vi "Read PID.vi"(7 "PIDs":T1, 8 "error in (no error)":errorcluster, 11 "VISA Refnum in":refnum<visa-resource-name>) -> (0 "error out":errorcluster, 2 "Response":string, 3 "Result":dbl format="%.2f")   [LabVIEW 2011]
uses:
  PID List.ctl
panel:
  out "number":u16
  out "length 2":i32
  out "sum":u32
  out "length":i32
  out "Serial Settings:Number of Bytes at Serial Port":u32
  out "read buffer 2":string
  out "read buffer":string
  out "Array":string[](array[string])
  out "Responses":string[](array[string])
  out "VISA Refnum in 2":refnum<visa-resource-name>
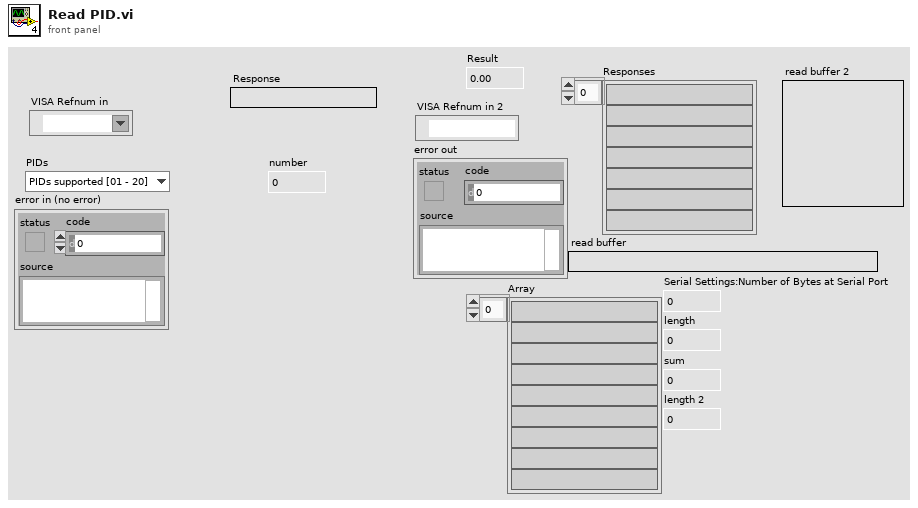
[diagram p1: front panel]
types:
  T1 = typedef "PID List.ctl" = enum16{"PIDs supported [01 - 20]", "Monitor status since DTCs cleared", "Freeze DTC", "Fuel system status", "Caulculated engine load value", "Engine Coolant temperature", "Short term fuel %trim Bank1", "Long term fuel %trim Bank 1", "Short term fuel %trim Bank2", "Long term fuel %trim Bank2", "Fuel pressure", "Intake manifold absolute pressure", "Engine RPM", "Vehicle speed", "timing advance", "Intake air temperature", "MAF air flow rate", "Throttle position", "Commanded secondary air status", "Oxygen sensors present", "bank 1 sensor 1", "Bank 1 sensor 2", "Bank 1 sensor 3", "Bank 1 sensor 4", "Bank 2 sensor 1", "Bank 2 sensor 2", "Bank 2 sensor 3", "Bank 2 sensor 4", "OBD standards this vehicle conforms to", "Oxygen sensor present", "Auxilary input status", "Run time since engine start", "PIDs supported [21-40]", "Distance traveled with malfunction", "Fuel Rail Pressure (manifold)", "Fuel Rail Pressure (gasoline)", "O2S1_WR", "O2S2_WR", "O2S3_WR", "O2S4_WR", "O2S5_WR", "O2S6_WR", "O2S7_WR", "O2S8_WR", "Commanded EGR", "EGR Error", "Commanded evaporative purge", "Fuel Level Input", "# of warm ups since codes cleared", "Distance traveled since codes cleared", "Evap System Vapor Pressure", "Barometric pressure", "O2S1", "O2S2", "O2S3", "O2S4", "O2S5", "O2S6", "O2S7", "O2S8", "Catalyst Temperature B1S1", "Catalyst Temperature B2S1", "Catalyst Temperature B1S2", "Catalyst Temperature B2S2", "PIDs supported [41-60]", "Monitor status this drive cycle", "Control module voltage", "Absolute load value", "Command equivalence ratio", "Relative throttle position", "Ambient air temperature", "Absolute throttle position B", "Absolute throttle position C", "Accelerator pedal position D", "Accelerator pedal position E", "Accelerator pedal position F", "Command throttle actuator", "PIDs supported [61-80]", "Auxilary input / output supported", "Mass air flow sensor", "Engine coolant temperature", "Intake air temperature sensor", "Commanded EGR and EGR Error", "Fuel pressure control system", "Injection pressure control system", "Turbocharger compressor inlet pressure", "Boost pressure control", "Exhaust pressure", "Turbocharger RPM", "Turbocharger temperature", "Turbocharger temperature2", "Vehicle Identification number (VIN)"}
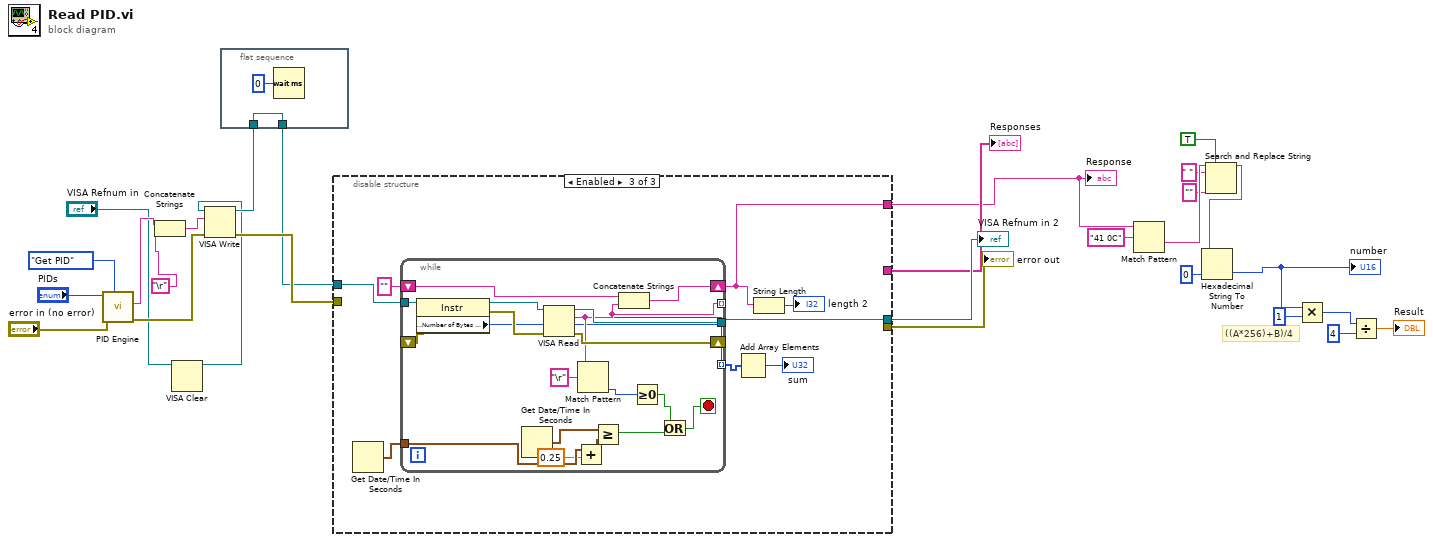
[diagram p0: block diagram]
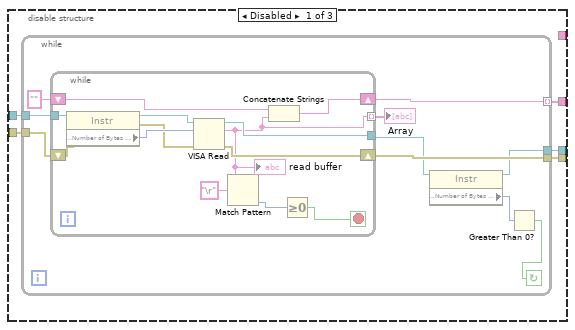
[diagram p2: hidden frame]
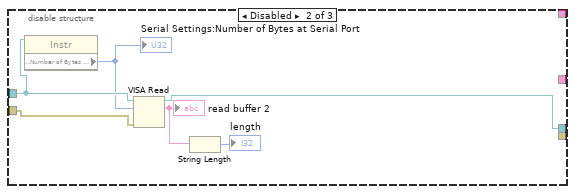
[diagram p3: hidden frame]
diagram:
  # "((A*256)+B)/4"
  n1 = call "PID Engine.vi"("State"=enum16{"Init", "Get PID"}."Get PID", "error in (no error)"="error in (no error)", "PIDs"="PIDs") -> ("error out"=w25:errorcluster, "String"=w22:string)  [unwired: 5 in, 2 out]
  n2 = Concatenate Strings(w22, "\r") -> (w21:string)
  n3 = VISA Clear(VISA resource name="VISA Refnum in") -> (VISA resource name out=w14:refnum<visa-resource-name>)  [unwired: 1 in, 1 out]
  n4 = VISA Write(VISA resource name=w14, write buffer=w21, error in (no error)=w25) -> (VISA resource name out=w16:refnum<visa-resource-name>, error out=w24:errorcluster)  [unwired: 1 out]
  n5 = flat-sequence {
    tunnel: [w29] -> w17
    tunnel: w16 -> [w29]
    frame #0 {
      n6 = Wait (ms)(milliseconds to wait=u32 0) -> ()  [unwired: 1 out]
    }
  }
  n7 = disable-structure shown="Enabled" {
    disable-tunnel: w24 -> [w35 w64 _]
    disable-tunnel: [w34 _ _] -> w23
    disable-tunnel: [w33 w63 w66] -> w19
    disable-tunnel: [w32 _ _] -> w18
    disable-tunnel: w17 -> [w31 w62 w71]
    disable-tunnel: [_ _ w67] -> w13
    frame Disabled {
      n8 = while {
        tunnel: w31 -> [w45]
        tunnel: [w43] -> w32 mode=indexing
        tunnel: w35 -> [w42]
        tunnel: [w41] -> w34
        tunnel: [w39] -> w33
        stop <- w37 continue-if-true
        n9 = while {
          tunnel: w45 -> [w58]
          shift-right: [w51] -> w43
          shift-left: "" -> [w50]
          tunnel: [w49] -> w40
          shift-right: [w48] -> w41
          shift-left: w42 -> [w47]
          tunnel: [w46] -> w36 mode=indexing
          stop <- w52 stop-if-true
          n10 = property class="Instr"(reference=w58, error in=w47) -> (reference out=w57:refnum<visa-resource-name>, error out=w55:errorcluster, "Serial Settings:Number of Bytes at Serial Port"=w56:u32)
          n11 = VISA Read(VISA resource name=w57, byte count=w56, error in (no error)=w55) -> (VISA resource name out=w49:refnum<visa-resource-name>, read buffer=w46:string, error out=w48:errorcluster)  [unwired: 1 out]
          "read buffer" <- w46
          n12 = Match Pattern(string=w46, regular expression="\r") -> (offset past match=w53:i32)  [unwired: 1 in, 3 out]
          n13 = Concatenate Strings(w50, w46) -> (w51:string)
          n14 = Greater Or Equal To 0?(x=w53) -> (x >= 0?=w52:bool)
        }
        "Array" <- w36
        n15 = property class="Instr"(reference=w40) -> (reference out=w39:refnum<visa-resource-name>, "Serial Settings:Number of Bytes at Serial Port"=w38:u32)  [unwired: 1 in, 1 out]
        n16 = Greater Than 0?(x=w38) -> (x > 0?=w37:bool)
      }
    }
    frame Disabled {
      n17 = property class="Instr"(reference=w62) -> ("Serial Settings:Number of Bytes at Serial Port"=w61:u32)  [unwired: 1 in, 2 out]
      "Serial Settings:Number of Bytes at Serial Port" <- w61
      n18 = VISA Read(VISA resource name=w62, byte count=w61, error in (no error)=w64) -> (VISA resource name out=w63:refnum<visa-resource-name>, read buffer=w60:string)  [unwired: 2 out]
      "read buffer 2" <- w60
      n19 = String Length(string=w60) -> (length=→"length":i32)
    }
    frame Enabled {
      n20 = Get Date/Time In Seconds() -> (seconds since 1Jan1904=w65:timestamp)
      n21 = while {
        tunnel: w71 -> [w91]
        shift-right: [w86] -> w67
        shift-left: "" -> [w85]
        tunnel: [w84] -> w66
        shift-right: [w83] -> _
        shift-left: _ -> [w82]
        tunnel: [w81] -> _ mode=indexing
        tunnel: [w80] -> w70 mode=indexing
        tunnel: w65 -> [w78]
        stop <- w74 stop-if-true
        n22 = property class="Instr"(reference=w91, error in=w82) -> (reference out=w90:refnum<visa-resource-name>, error out=w89:errorcluster, "Serial Settings:Number of Bytes at Serial Port"=w80:u32)
        n23 = Get Date/Time In Seconds() -> (seconds since 1Jan1904=w79:timestamp)
        n24 = VISA Read(VISA resource name=w90, byte count=w80, error in (no error)=w89) -> (VISA resource name out=w84:refnum<visa-resource-name>, read buffer=w81:string, error out=w83:errorcluster)  [unwired: 1 out]
        n25 = Add(x=w78, y=0.25) -> (x+y=w76:timestamp)
        n26 = Match Pattern(string=w81, regular expression="\r") -> (offset past match=w87:i32)  [unwired: 1 in, 3 out]
        n27 = Greater Or Equal?(x=w79, y=w76) -> (x >= y?=w73:bool)
        n28 = Concatenate Strings(w85, w81) -> (w86:string)
        n29 = Greater Or Equal To 0?(x=w87) -> (x >= 0?=w75:bool)
        n30 = Or(x=w75, y=w73) -> (x .or. y?=w74:bool)
      }
      n31 = Add Array Elements(numeric array=w70) -> (sum=→"sum":u32)
      n32 = String Length(string=w67) -> (length=→"length 2":i32)
    }
  }
  "Response" <- w13
  "VISA Refnum in 2" <- w19
  "error out" <- w23
  "Responses" <- w18
  n33 = Match Pattern(string=w13, regular expression="41 0C") -> (after substring=w10:string)  [unwired: 1 in, 3 out]
  n34 = Search and Replace String(replace all?=TRUE ("replace all? (F)"), input string=w10, search string=" ", replace string="" ("replace string (\"\")")) -> (result string=w9:string)  [unwired: 4 in, 3 out]
  n35 = Hexadecimal String To Number(string=w9, default (0uL)=u16 0 ("default (0 U32)")) -> (number=w5:u16)  [unwired: 1 in, 1 out]
  "number" <- w5
  n36 = Multiply(x=w5, y=u16 1) -> (x*y=w3:u16)
  n37 = Divide(x=w3, y=u16 4) -> (x/y=→"Result":dbl)
